vi "Configure Colors.vi"(0 "Current Color":T1) -> (1 "Array":cluster{"FG":u32, "BG":u32}[](array[cluster]), 2 "Text Colors":T2)   [LabVIEW 2012, in "Hover Button.xctl"]
doc: "This vi converts a color set from the State data to the format needed to write to the Boolean button properties."
uses:
  Hover Button.xctl
  Button Colors.ctl
panel:
  # "This vi reads in the color related State data\nand converts it to the format required for\nthe Boolean button properties"
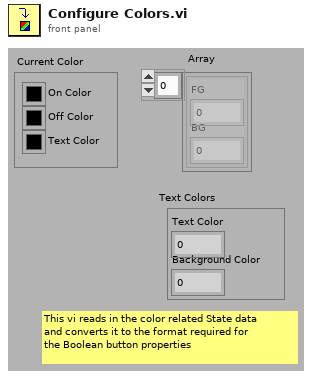
[diagram p1: front panel]
types:
  T1 = typedef "Hover Button.xctl/Button Colors.ctl" = cluster{"On Color":u32, "Text Color":u32, "Off Color":u32}
  T2 = cluster{"Text Color":u32, "Background Color":u32}
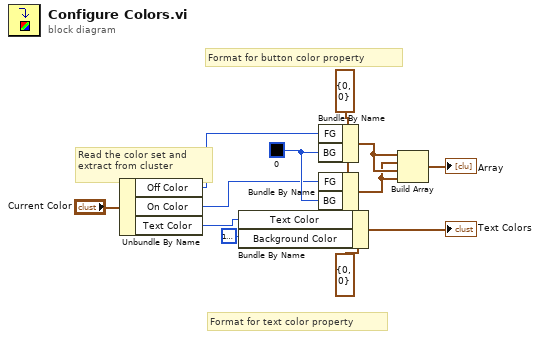
[diagram p0: block diagram]
diagram:
  w6 = cluster{"FG":u32, "BG":u32} {"FG"=0, "BG"=0}
  w5 = u32 0
  # "Format for button color property"
  # "Format for text color property"
  # "Read the color set and\nextract from cluster"
  n1 = Unbundle By Name("Current Color") -> ("Off Color"=w7:u32, "On Color"=w4:u32, "Text Color"=w10:u32)
  n2 = Bundle By Name(cluster=T2 {"Text Color"=0, "Background Color"=0} ("Boolean Text.Text Colors"), "Text Color"=w10, "Background Color"=u32 16777216) -> (→"Text Colors":T2)
  n3 = Bundle By Name(cluster=w6, "FG"=w7, "BG"=w5) -> (w2:cluster{"FG":u32, "BG":u32})
  n4 = Bundle By Name(cluster=w6, "FG"=w4, "BG"=w5) -> (w1:cluster{"FG":u32, "BG":u32})
  n5 = Build Array(w2, w1, w2, w1) -> (→"Array":cluster{"FG":u32, "BG":u32}[])
